vi "reset_button.vi"(10 "字符串":string, 11 "Cluster输入":refnum<vi>) -> (3 "Cluster输入 2":refnum<vi>)   [LabVIEW 2018, in "UI.lvlib"]
uses:
  UI.lvlib
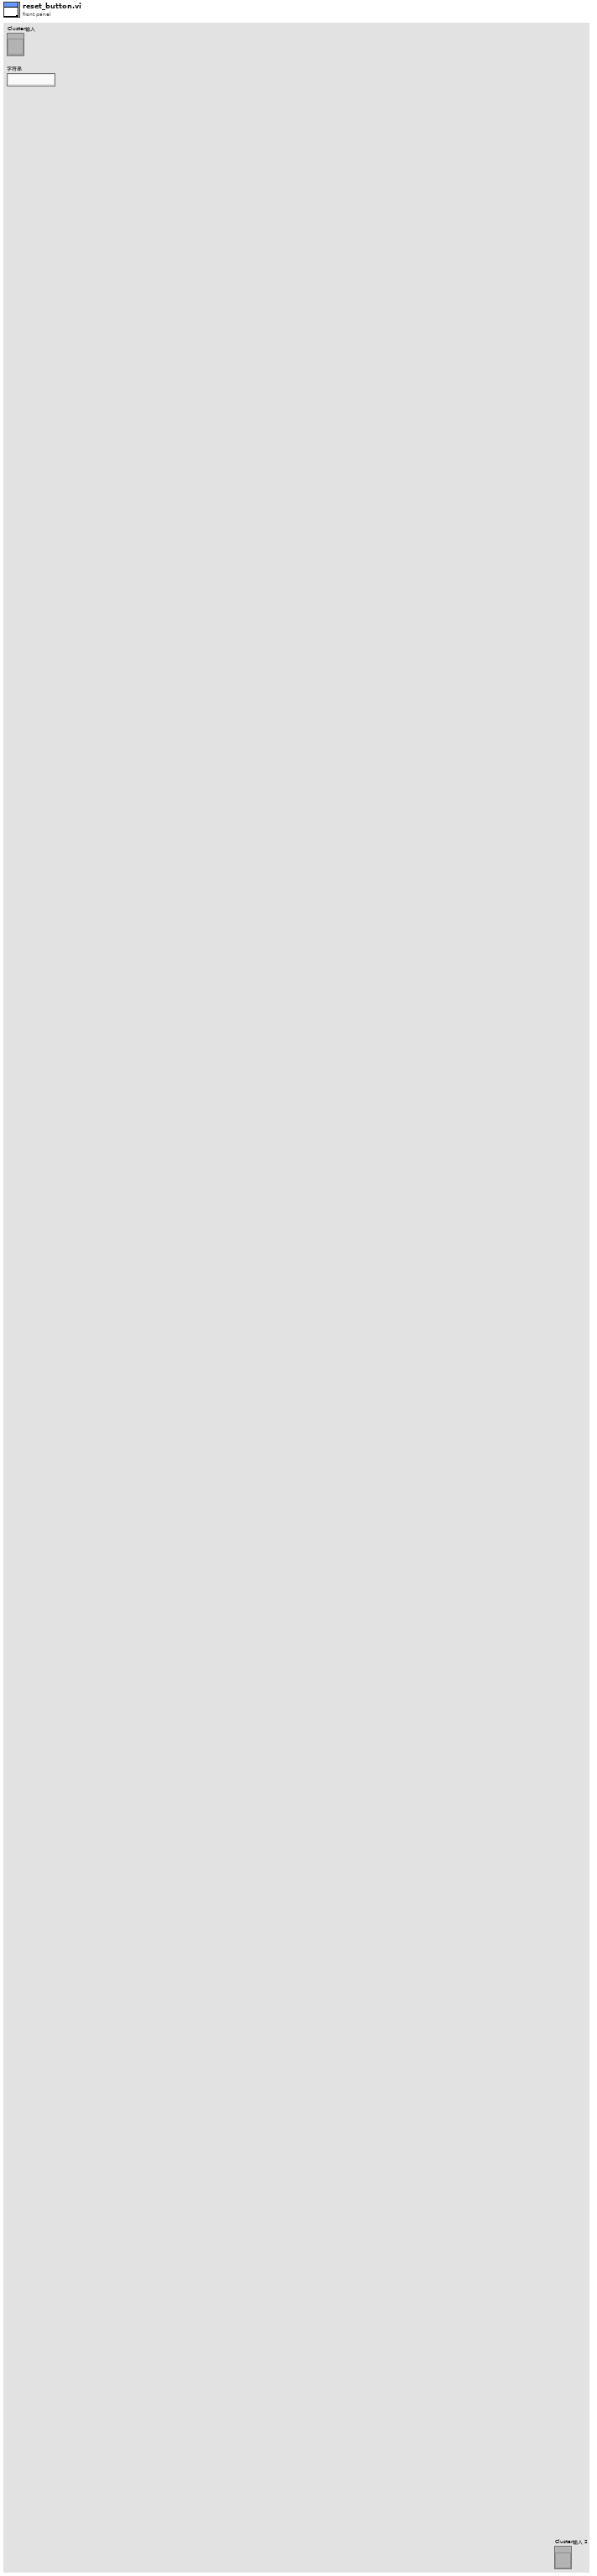
[diagram p1: front panel]
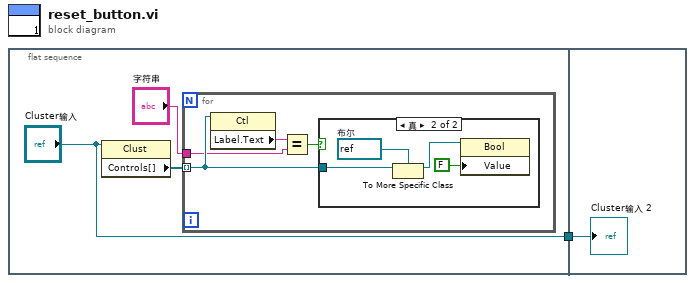
[diagram p0: block diagram]
diagram:
  n1 = flat-sequence {
    tunnel: ["Cluster输入"] -> w1
    tunnel: w1 -> [w13]
    frame #0 {
      n2 = property class="Clust"(reference="Cluster输入") -> ("Controls[]"=w4:refnum<vi>[])  [unwired: 1 in, 2 out]
      n3 = for {
        tunnel: w4 -> [w8] mode=indexing
        tunnel: "字符串" -> [w6]
        n4 = property class="Ctl"(reference=w8) -> ("Label.Text"=w7:string)  [unwired: 1 in, 2 out]
        n5 = Equal?(x=w7, y=w6) -> (x = y?=w5:bool)
        n6 = case shown="真" w5 {
          tunnel: w8 -> [_ w12]
          frame False {
          }
          frame True {
            w11 = refnum<vi> refnum  # 布尔
            n7 = To More Specific Class(target class=w11, reference=w12) -> (specific class reference=w10:refnum<vi>)  [unwired: 1 in, 1 out]
            n8 = property class="Bool"(reference=w10, "Value"=FALSE) -> ()  [unwired: 1 in, 2 out]
          }
        }
      }
    }
    frame #1 {
      "Cluster输入 2" <- w13
    }
  }
